vi "Trace_Inspector.vi"() -> ()   [LabVIEW 2010]
uses:
  <vilib>/Utility/file.llb/Read From Spreadsheet File (DBL).vi
  <vilib>/Analysis/NI_AALBase.lvlib
panel:
  in  "Dummyzoomthis":bool
  in  "Display mode":enum32{"Raw", "DF/F"}(radio)
  out "F0":dbl
  in  "SetF0":bool
  out "Loading":bool
  in  "file path (dialog if empty)":path
  out "Current file":path
  in  "Boxcar pixels":i32=1 min=1 max=10000 step=1
  in  "Postprocessing":enum32{"Unfiltered", "Filtered"}(radio)
  in  "Zoom_this":bool
  out "Zoom graph":cluster{"X":dbl, dbl, dbl[]}(graph)
  out "Total graph":cluster{dbl, dbl, "Data out":dbl[]}(graph)
  in  "Channel selection":enum32{"Channel 1", "Channel 2", "Channel 3"}(radio)
  in  "Quit":bool
  in  "Open":bool
  # "Fiber - fMRI\nTrace inspector"
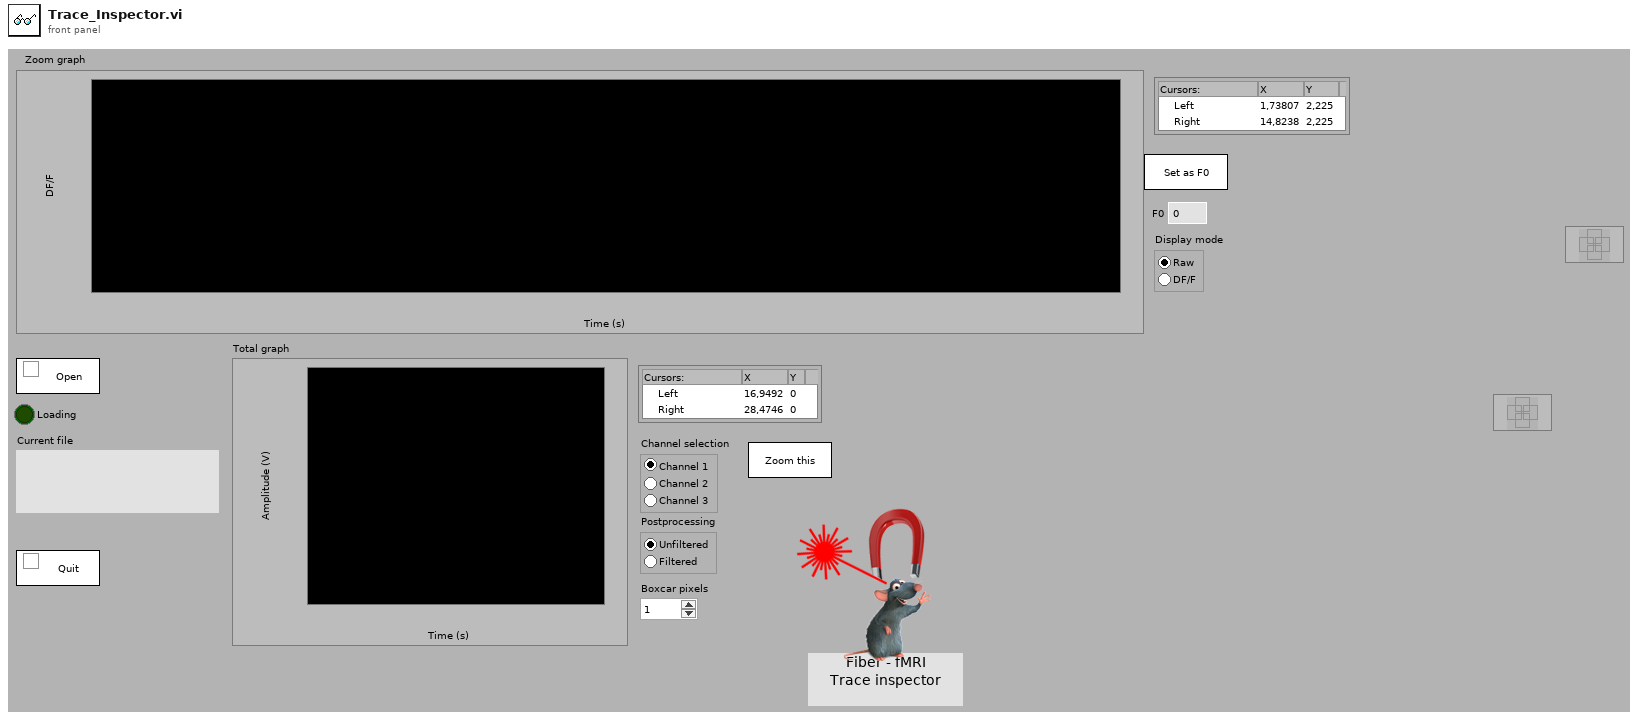
[diagram p1: front panel]
types:
  T1 = typedef "LVCursorListTypeDef.ctl" = cluster{"Name":string, "Color":u32, "Style":u8, "Point Style":u8, "Name Visible":bool, "Allow Drag":bool, "Cursor Mode":u32, "Plot":i32, "Index":i32, "Position":cluster{"X":dbl, "Y":dbl}, "X Scale":u32, "Y Scale":u32, "Watch Plots":i32[], "Watch All Plots":bool, "Plot Area":i32, "Label Offset":cluster{"X":dbl, "Y":dbl}}[]
  T2 = cluster{"Name":string, "Color":u32, "Style":u8, "Point Style":u8, "Name Visible":bool, "Allow Drag":bool, "Cursor Mode":u32, "Plot":i32, "Index":i32, "Position":cluster{"X":dbl, "Y":dbl}, "X Scale":u32, "Y Scale":u32, "Watch Plots":i32[], "Watch All Plots":bool, "Plot Area":i32, "Label Offset":cluster{"X":dbl, "Y":dbl}}
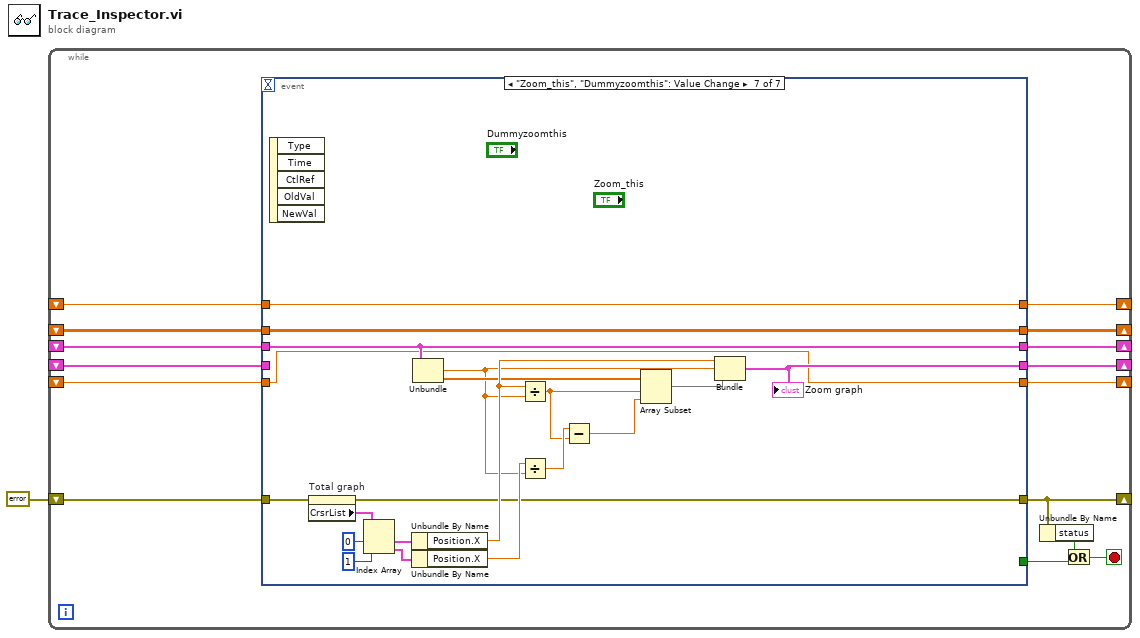
[diagram p0: block diagram]
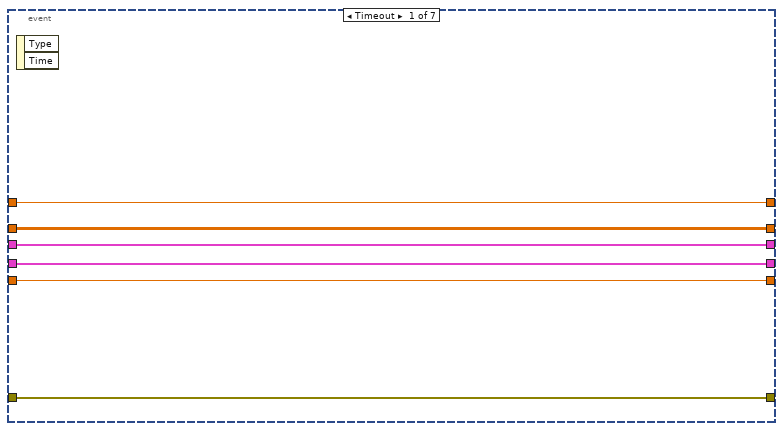
[diagram p2: hidden frame]
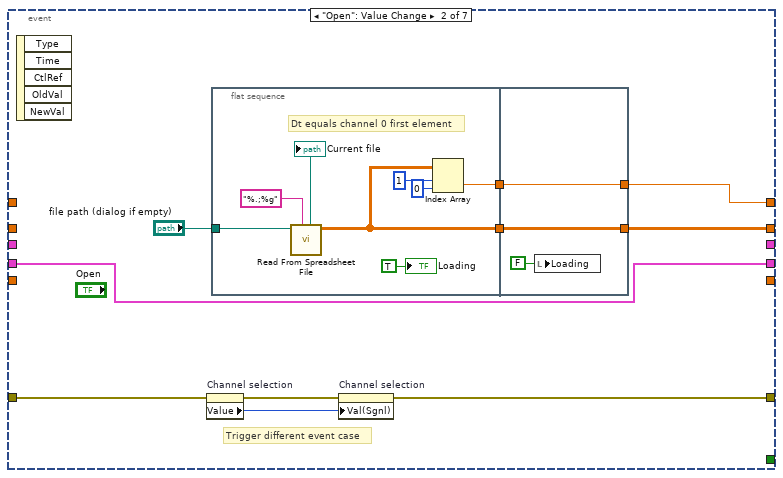
[diagram p3: hidden frame]
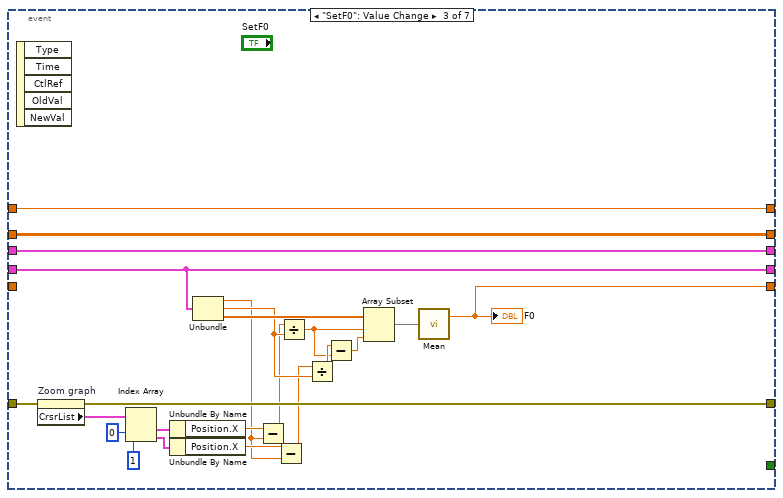
[diagram p4: hidden frame]
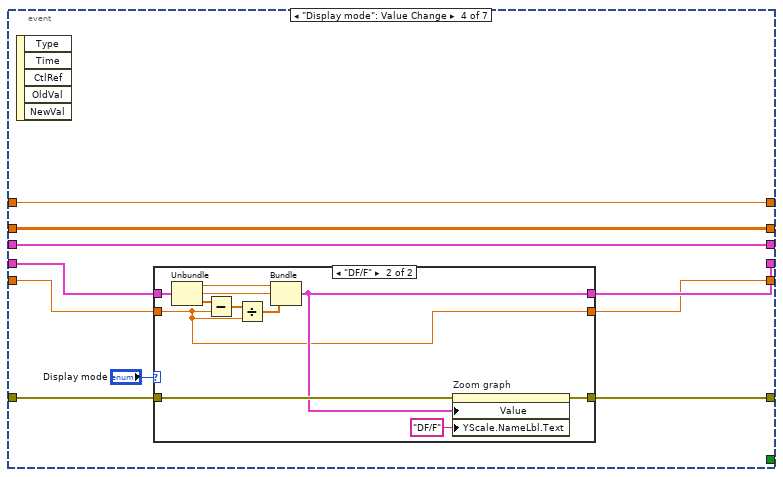
[diagram p5: hidden frame]
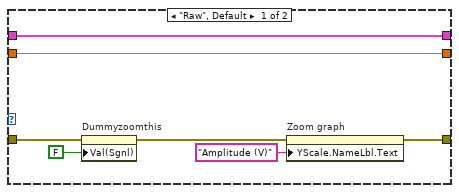
[diagram p6: hidden frame]
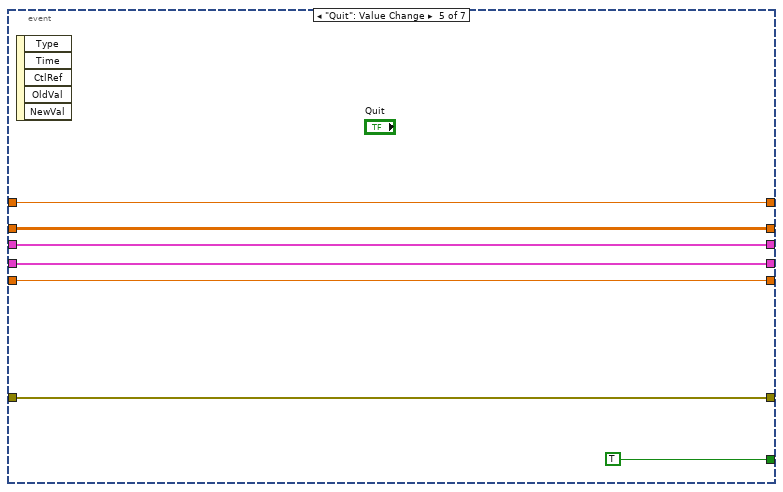
[diagram p7: hidden frame]
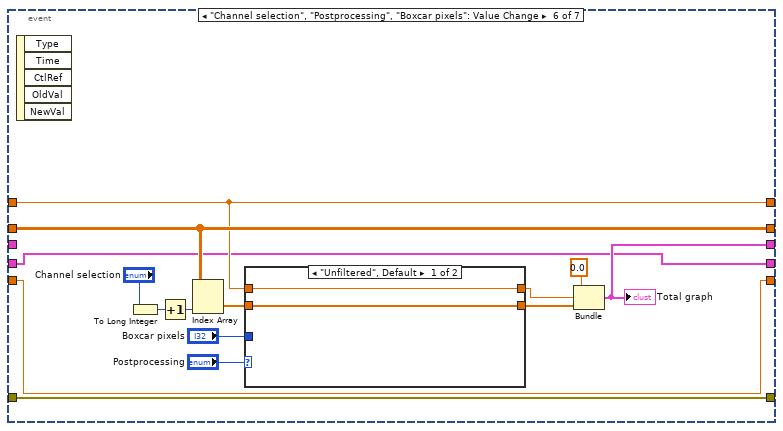
[diagram p8: hidden frame]
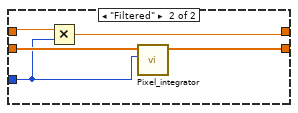
[diagram p9: hidden frame]
diagram:
  n1 = while {
    shift-right: [w15] -> _
    shift-left: errorcluster {"status"=FALSE, "code"=0, "source"=""} ("error in") -> [w16]
    shift-right: [w11] -> _
    shift-left: _ -> [w10]
    shift-right: [w9] -> _
    shift-left: _ -> [w8]
    shift-right: [w7] -> _
    shift-left: _ -> [w6]
    shift-right: [w5] -> _
    shift-left: _ -> [w4]
    shift-right: [w3] -> _
    shift-left: _ -> [w2]
    stop <- w12 stop-if-true
    n2 = event shown="[6] \"Zoom_this\", \"Dummyzoomthis\": Value Change" {
      selector: _ -> [_ _ _ _ _ _ _]
      dyn-events: _ -> [_ _ _ _ _ _ _]
      timeout: _ -> [_ _ _ _ _ _ _]
      tunnel: w16 -> [w22 w31 w64 w74 w101 w116 w143]
      tunnel: [w22 w30 w51 w73 w101 w116 w124] -> w15
      tunnel: [_ _ _ _ TRUE _ _] -> w13
      tunnel: [w20 w28 w65 w69 w97 w112 w137] -> w11
      tunnel: w10 -> [w20 _ w65 w69 w97 w112 w137]
      tunnel: [w21 _ w44 w68 w96 w110 w130] -> w9
      tunnel: w8 -> [w21 _ w44 w68 w96 _ w130]
      tunnel: [w19 w27 w66 w76 w99 w105 w128] -> w7
      tunnel: w6 -> [w19 _ w66 w76 w99 w105 w128]
      tunnel: [w18 w23 w52 w71 w98 w103 w126] -> w5
      tunnel: w4 -> [w18 w23 w52 w72 w98 w103 _]
      tunnel: [w17 _ w50 w67 w95 w102 w125] -> w3
      tunnel: w2 -> [w17 _ _ w70 w95 w102 w125]
      event Timeout {
        n3 = event-data() -> ()  [unwired: 1 in, 2 out]
      }
      event "Open": Value Change {
        # "Trigger different event case"
        n4 = event-data() -> ()  [unwired: 1 in, 5 out]
        n5 = property on="Channel selection" class="RadioBtnsControl (strict)"(error in=w31) -> (error out=w32:errorcluster, "Value"=w29:enum32{"Channel 1", "Channel 2", "Channel 3"})  [unwired: 1 in, 1 out]
        n6 = flat-sequence {
          tunnel: "file path (dialog if empty)" -> [w34]
          tunnel: [w37] -> w25
          tunnel: [w36] -> w24
          tunnel: [w42] -> w27
          tunnel: [w43] -> w28
          tunnel: w25 -> [w43]
          tunnel: w24 -> [w42]
          frame #0 {
            # "Dt equals channel 0 first element"
            n7 = call-poly <vilib>:"Read From Spreadsheet File.vi"("format (%.3f)"="%.;%g", "file path (dialog if empty)"=w34) -> ("all rows"=w37:dbl[][], "new file path (Not A Path if cancelled)"=→"Current file":path)  [unwired: 5 in, 3 out]
            n8 = Index Array(array=w37, index (row)=1 ("disabled index (row)"), index (col)=0 ("disabled index (col)")) -> (element=w36:dbl)
            "Loading" <- TRUE ("Loading")
          }
          frame #1 {
            n9 = local write "Loading"(FALSE ("Loading")) -> ()
          }
        }
        n10 = property on="Channel selection" class="RadioBtnsControl (strict)"(error in=w32, "Val(Sgnl)"=w29) -> (error out=w30:errorcluster)  [unwired: 1 in, 1 out]
      }
      event "SetF0": Value Change {
        n11 = event-data() -> ()  [unwired: 1 in, 5 out]
        n12 = property on="Zoom graph" class="WFGraph (strict)"(error in=w64) -> (error out=w51:errorcluster, "CrsrList"=w63:T1)  [unwired: 1 in, 1 out]
        n13 = Index Array(array=w63, index #1=0 ("index"), index #2=1 ("index")) -> (element #1=w60:T2, element #2=w59:T2)
        n14 = Unbundle By Name(w60) -> ("Position.X"=w49:dbl)
        n15 = Unbundle By Name(w59) -> ("Position.X"=w48:dbl)
        n16 = Unbundle(w52) -> ("X"=w47:dbl, w57:dbl, w58:dbl[])
        n17 = Subtract(x=w49, y=w47) -> (x-y=w46:dbl)
        n18 = Subtract(x=w48, y=w47) -> (x-y=w45:dbl)
        n19 = Divide(x=w46, y=w57) -> (x/y=w55:dbl)
        n20 = Divide(x=w45, y=w57) -> (x/y=w56:dbl)
        n21 = Subtract(x=w56, y=w55) -> (x-y=w54:dbl)
        n22 = Array Subset(array=w58, index=w55, length=w54) -> (w53:dbl[])
        n23 = call <vilib>:"Mean.vi"("X"=w53) -> ("mean"=w50:dbl)  [unwired: 1 out]
        "F0" <- w50
      }
      event "Display mode": Value Change {
        n24 = event-data() -> ()  [unwired: 1 in, 5 out]
        n25 = case shown="\"DF/F\"" "Display mode" {
          tunnel: [w79 w87] -> w73
          tunnel: w74 -> [w82 w88]
          tunnel: w72 -> [w83 w94]
          tunnel: w70 -> [w77 w84]
          tunnel: [w83 w86] -> w71
          tunnel: [w77 w84] -> w67
          frame "Raw", Default {
            n26 = property on="Dummyzoomthis" class="Bool (strict)"(error in=w82, "Val(Sgnl)"=FALSE) -> (error out=w80:errorcluster)  [unwired: 1 in, 1 out]
            n27 = property on="Zoom graph" class="WFGraph (strict)"(error in=w80, "YScale.NameLbl.Text"="Amplitude (V)" ("Y Scale.Name Label.Text")) -> (error out=w79:errorcluster)  [unwired: 1 in, 1 out]
          }
          frame "DF/F" {
            n28 = Unbundle(w94) -> ("X"=w91:dbl, w90:dbl, w93:dbl[])
            n29 = Subtract(x=w93, y=w84) -> (x-y=w92:dbl[])
            n30 = Divide(x=w92, y=w84) -> (x/y=w89:dbl[])
            n31 = Bundle("X"=w91, w90, w89) -> (w86:cluster{"X":dbl, dbl, dbl[]})  [unwired: 1 in]
            n32 = property on="Zoom graph" class="WFGraph (strict)"(error in=w88, "Value"=w86, "YScale.NameLbl.Text"="DF/F" ("Y Scale.Name Label.Text")) -> (error out=w87:errorcluster)  [unwired: 1 in, 1 out]
          }
        }
      }
      event "Quit": Value Change {
        n33 = event-data() -> ()  [unwired: 1 in, 5 out]
      }
      event "Channel selection", "Postprocessing", "Boxcar pixels": Value Change {
        n34 = event-data() -> ()  [unwired: 1 in, 5 out]
        n35 = To Long Integer(number="Channel selection") -> (32bit integer=w113:i32)
        n36 = Increment(x=w113) -> (x+1=w115:i32)
        n37 = Index Array(array=w112, index (col)=w115) -> (element=w108:dbl[])  [unwired: 1 in]
        n38 = case shown="\"Unfiltered\", Default" "Postprocessing" {
          tunnel: [w118 w122] -> w107
          tunnel: w108 -> [w118 w123]
          tunnel: "Boxcar pixels" -> [_ w120]
          tunnel: w105 -> [w117 w121]
          tunnel: [w117 w119] -> w104
          frame "Unfiltered", Default {
          }
          frame "Filtered" {
            n39 = Multiply(x=w121, y=w120) -> (x*y=w119:dbl)
            n40 = call "Pixel_integrator.vi"("Pixels to integrate"=w120, "Data in"=w123) -> ("Data out"=w122:dbl[])  [unwired: 6 in, 1 out]
          }
        }
        n41 = Bundle(0.0, w104, "Data out"=w107) -> (w110:cluster{dbl, dbl, "Data out":dbl[]})  [unwired: 1 in]
        "Total graph" <- w110
      }
      event "Zoom_this", "Dummyzoomthis": Value Change {
        n42 = event-data() -> ()  [unwired: 1 in, 5 out]
        n43 = property on="Total graph" class="WFGraph (strict)"(error in=w143) -> (error out=w124:errorcluster, "CrsrList"=w142:T1)  [unwired: 1 in, 1 out]
        n44 = Index Array(array=w142, index #1=0 ("index"), index #2=1 ("index")) -> (element #1=w141:T2, element #2=w138:T2)
        n45 = Unbundle By Name(w141) -> ("Position.X"=w132:dbl)
        n46 = Unbundle By Name(w138) -> ("Position.X"=w136:dbl)
        n47 = Unbundle(w130) -> (w127:dbl, "Data out"=w129:dbl[])  [unwired: 1 out]
        n48 = Divide(x=w132, y=w127) -> (x/y=w134:dbl)
        n49 = Divide(x=w136, y=w127) -> (x/y=w135:dbl)
        n50 = Subtract(x=w135, y=w134) -> (x-y=w133:dbl)
        n51 = Array Subset(array=w129, index=w134, length=w133) -> (w131:dbl[])
        n52 = Bundle("X"=w132, w127, w131) -> (w126:cluster{"X":dbl, dbl, dbl[]})  [unwired: 1 in]
        "Zoom graph" <- w126
      }
    }
    n53 = Unbundle By Name(w15) -> ("status"=w14:bool)
    n54 = Or(x=w14, y=w13) -> (x .or. y?=w12:bool)
  }
